vi "Configure RJDJ Extraction Characteristics.vi"(0 "VISA resource name":refnum<visa-resource-name>, 1 "Jitter Removal (0: On)":i32(ring) items=["On", "Auto", "Off"], 2 "Jitter to Remove (300e-15)":dbl=3e-13, 5 "Random Jitter Method (0: Spectral)":i32(ring) items=["Spectral", "Both"], 7 "Report Method (0: Spectral)":i32(ring) items=["Spectral", "Tail Fit"], 9 "Enable Specified Jitter (F: Disable)":bool, 11 "error in (no error)":errorcluster, 12 "Random Jitter (0)":dbl) -> (4 "VISA resource name out":refnum<visa-resource-name>, 15 "error out":errorcluster)   [LabVIEW 2020, in "Agilent 90000 Series.lvlib"]
doc: "Configures settings for Random Jitter (RJ) and Deterministic Jitter (DJ)."
uses:
  Agilent 90000 Series.lvlib
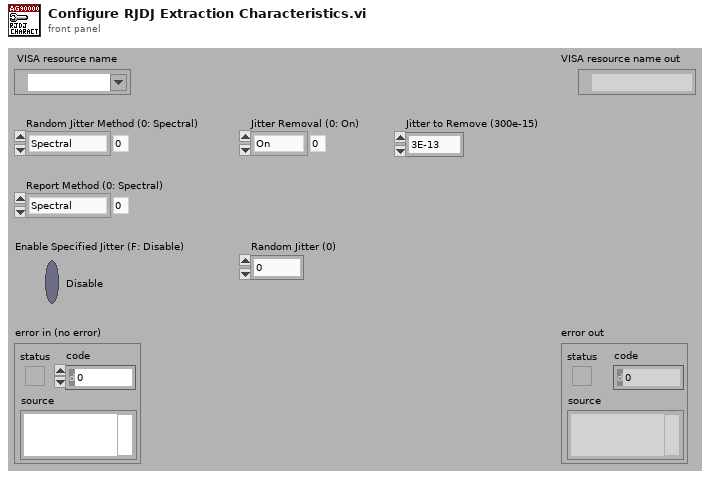
[diagram p1: front panel]
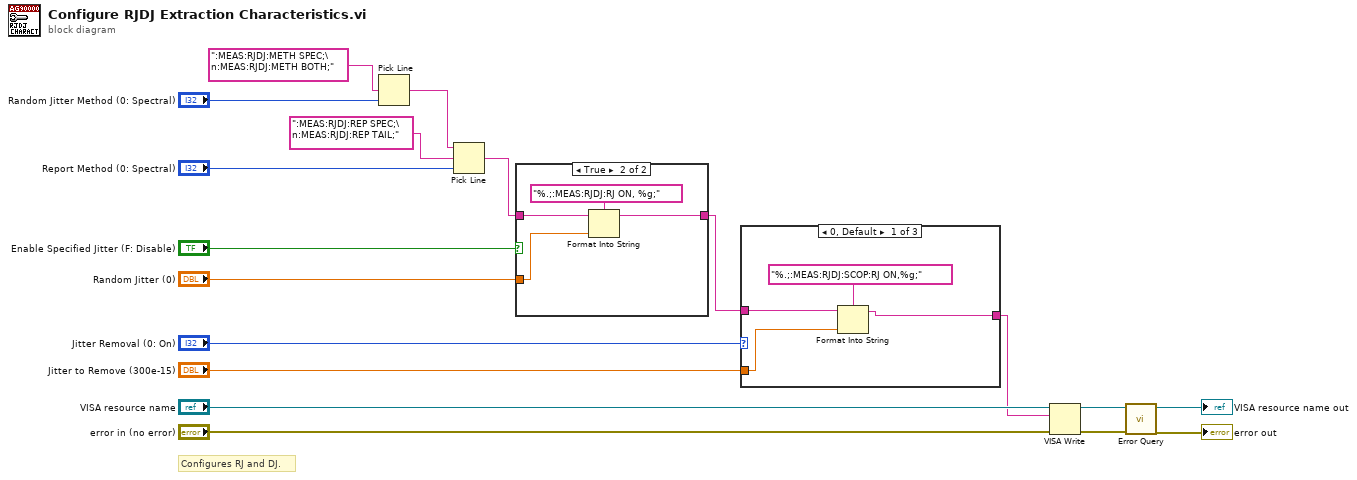
[diagram p0: block diagram]
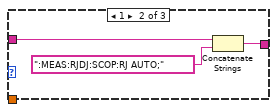
[diagram p2: hidden frame]
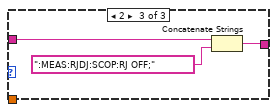
[diagram p3: hidden frame]
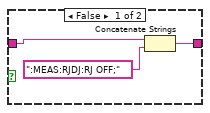
[diagram p4: hidden frame]
diagram:
  # "Configures RJ and DJ."
  n1 = Pick Line(multi-line string=":MEAS:RJDJ:METH SPEC;\n:MEAS:RJDJ:METH BOTH;", line index="Random Jitter Method (0: Spectral)") -> (output string=w14:string)  [unwired: 1 out]
  n2 = Pick Line(string ("")=w14, multi-line string=":MEAS:RJDJ:REP SPEC;\n:MEAS:RJDJ:REP TAIL;", line index="Report Method (0: Spectral)") -> (output string=w6:string)
  n3 = case shown="True" "Enable Specified Jitter (F: Disable)" {
    tunnel: w6 -> [w20 w25]
    tunnel: [w21 w23] -> w3
    tunnel: "Random Jitter (0)" -> [_ w22]
    frame False {
      n4 = Concatenate Strings(w20, ":MEAS:RJDJ:RJ OFF;") -> (w21:string)
    }
    frame True {
      n5 = Format Into String(format string="%.;:MEAS:RJDJ:RJ ON, %g;", initial string=w25, w22) -> (resulting string=w23:string)  [unwired: 1 in, 1 out]
    }
  }
  n6 = case shown="0, Default" "Jitter Removal (0: On)" {
    tunnel: w3 -> [w28 w32 w35]
    tunnel: [w27 w30 w33] -> w1
    tunnel: "Jitter to Remove (300e-15)" -> [w26 _ _]
    frame 0, Default {
      n7 = Format Into String(format string="%.;:MEAS:RJDJ:SCOP:RJ ON,%g;", initial string=w28, w26) -> (resulting string=w27:string)  [unwired: 1 in, 1 out]
    }
    frame 1 {
      n8 = Concatenate Strings(w32, ":MEAS:RJDJ:SCOP:RJ AUTO;") -> (w30:string)
    }
    frame 2 {
      n9 = Concatenate Strings(w35, ":MEAS:RJDJ:SCOP:RJ OFF;") -> (w33:string)
    }
  }
  n10 = VISA Write(VISA resource name="VISA resource name", write buffer=w1, error in (no error)="error in (no error)") -> (VISA resource name out=w11:refnum<visa-resource-name>, error out=w10:errorcluster)  [unwired: 1 out]
  n11 = call "Error Query.vi"("error in (no error)"=w10, "VISA resource name"=w11) -> ("error out"=→"error out":errorcluster, "VISA resource name out"=→"VISA resource name out":refnum<visa-resource-name>)  [unwired: 8 out]
